vi "initialize core.vi"(8 "error in":errorcluster, 9 "handler properties":T1={"max url size"=8000, "max header"=8000, "timeout ms"=5000, "max data size"=104857600}, 10 "connection handler pool size":i32=10, 11 "port":u16=80) -> (0 "error out":errorcluster, 3 "Basic HTTP server out":refnum<class "Basic HTTPS server.lvclass">)   [LabVIEW 2016, in "Basic HTTPS server.lvclass"]
uses:
  Basic HTTPS server.lvclass
  http server properties.ctl
  http handler ref.ctl
  Basic HTTPS server.lvclass/Basic HTTPS server.ctl
  HTTP responder/https responder.lvclass
  HTTP handler dataset/HTTPS handler dataset.lvclass
  lvlibtls/server/lvlibretls server listener.lvclass
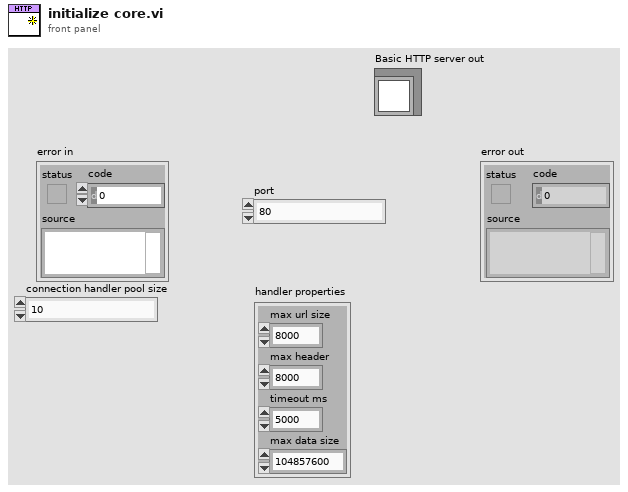
[diagram p1: front panel]
types:
  T1 = typedef "Basic HTTPS server.lvclass/http server properties.ctl" = cluster{"max url size":i32, "max header":i32, "timeout ms":i32, "max data size":i32}
  T2 = typedef "Basic HTTPS server.lvclass/http handler ref.ctl" = refnum<vi>
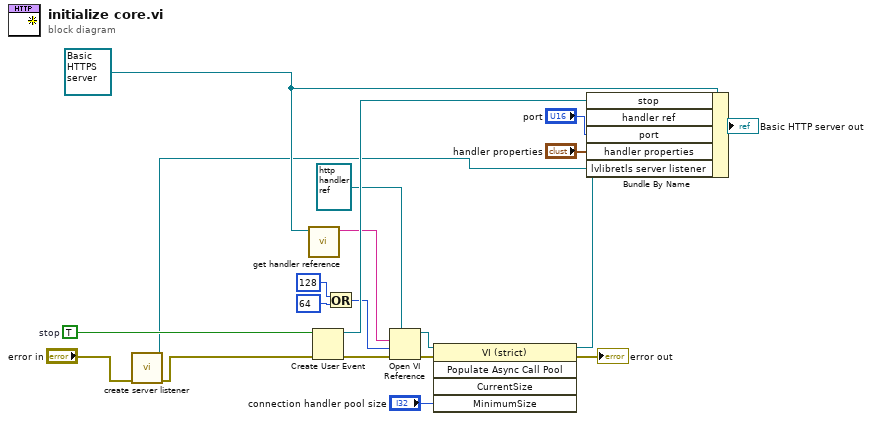
[diagram p0: block diagram]
diagram:
  w5 = refnum<class "Basic HTTPS server.lvclass"> refnum ("specialization")
  w20 = TRUE  # stop
  n1 = call "create server listener.vi"("error in"="error in") -> ("error out"=w2:errorcluster, "lvlibretls server listener out"=w1:refnum<class "lvlibretls server listener.lvclass">)  [unwired: 9 in]
  n2 = call "get handler reference.vi"("Basic HTTP server.lvclass"=w5) -> ("VI Name"=w4:string)  [unwired: 10 in]
  n3 = Create User Event(user event datatype=w20, error in=w2) -> (user event=w18:refnum<user-event>, error out=w17:errorcluster)
  n4 = Or(x=128 ("options"), y=64 ("options")) -> (x .or. y?=w15:i32)
  n5 = Open VI Reference(type specifier VI Refnum (for type only)=T2 refnum ("type"), vi path=w4, options=w15, error in (no error)=w17) -> (vi reference=w13:T2, error out=w16:errorcluster)  [unwired: 2 in]
  n6 = invoke class="VI (strict)" method="Populate Async Call Pool"(reference=w13, error in=w16, "MinimumSize"="connection handler pool size") -> (reference out=w9:T2, error out=→"error out":errorcluster)  [unwired: 2 in, 3 out]
  n7 = Bundle By Name(cluster=w5, "stop"=w18, "handler ref"=w9, "port"="port", "handler properties"="handler properties", "lvlibretls server listener"=w1) -> (→"Basic HTTP server out":refnum<class "Basic HTTPS server.lvclass">)
